vi "Read.vi"() -> (1 "Read Number":dbl=29.976272044892692, 2 "Read Location":string)   [LabVIEW 2023]
uses:
  <vilib>/OPCUA/client/Multiple Read Double.vi
  <vilib>/OPCUA/client/Multiple Read String.vi
  <vilib>/OPCUA/NI OPC UA Client.lvlib
panel:
  in  "Location Item Path":string="ns=2;s=Location.Location"
  in  "Data Item Path":string="ns=2;s=Data.Temperature"
  in  "Server Endpoint URL":string="opc.tcp://Beist:49580"
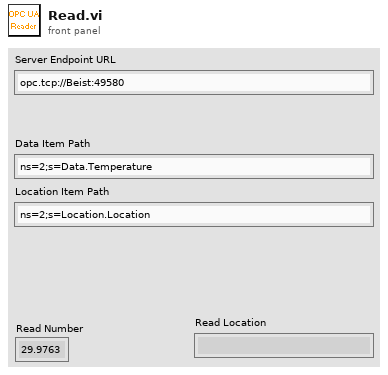
[diagram p1: front panel]
types:
  T1 = cluster{"message mode":enum16{"None", "Sign", "Sign and Encrypt"}, "security":enum16{"Basic256", "Basic128Rsa15"}}
  T2 = typedef "OPC UA Client Refnum.ctl" = refnum<k21>
  T3 = typedef "NodeId.ctl" = string
  T4 = typedef "OPC UA StatusCode.ctl" = u32
  T5 = cluster{"node ID":T3, "value ":dbl, "timestamp":timestamp, "status":T4}[]
  T6 = cluster{"node ID":T3, "value ":dbl, "timestamp":timestamp, "status":T4}
  T7 = cluster{"node ID":T3, "value ":string, "timestamp":timestamp, "status":T4}[]
  T8 = cluster{"node ID":T3, "value ":string, "timestamp":timestamp, "status":T4}
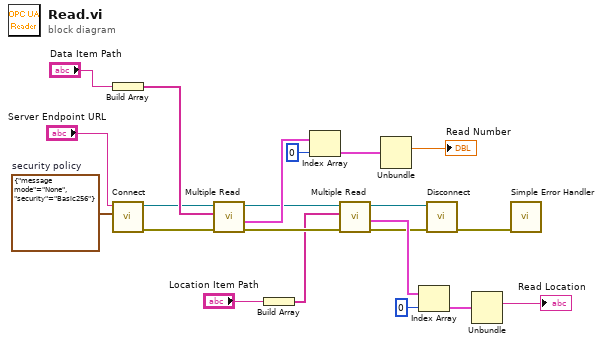
[diagram p0: block diagram]
diagram:
  w20 = T1 {"message mode"=enum."None", "security"=enum."Basic256"}  # security policy
  n1 = Build Array "Build Array"("Data Item Path") -> (w15:string[])
  n2 = call <vilib>:"Connect.vi"("security policy"=w20, "server endpoint URL"="Server Endpoint URL") -> ("error out"=w12:errorcluster, "OPC UA client refnum out"=w11:T2)  [unwired: 7 in, 1 out]
  n3 = call-poly <vilib>:"Multiple Read.vi"("error in (no error)"=w12, "node IDs"=w15, "OPC UA client refnum in"=w11) -> ("error out"=w5:errorcluster, "results"=w16:T5, "OPC UA client refnum out"=w6:T2)  [unwired: 5 in, 1 out]
  n4 = Build Array "Build Array"("Location Item Path") -> (w1:string[])
  n5 = Index Array "Index Array"(array=w16, index=0) -> (element=w17:T6)
  n6 = call-poly <vilib>:"Multiple Read.vi"("error in (no error)"=w5, "node IDs"=w1, "OPC UA client refnum in"=w6) -> ("error out"=w3:errorcluster, "results"=w7:T7, "OPC UA client refnum out"=w4:T2)  [unwired: 5 in, 1 out]
  n7 = Unbundle "Unbundle"(w17) -> ("value"=→"Read Number":dbl)  [unwired: 3 out]
  n8 = Index Array "Index Array"(array=w7, index=0) -> (element=w10:T8)
  n9 = call <vilib>:"Disconnect.vi"("error in (no error)"=w3, "OPC UA client refnum in"=w4) -> ("error out"=w19:errorcluster)  [unwired: 9 in]
  n10 = Unbundle "Unbundle"(w10) -> ("value"=→"Read Location":string)  [unwired: 3 out]
  n11 = call <vilib>:"Simple Error Handler.vi"("error in (no error)"=w19) -> ()  [unwired: 4 in, 5 out]
